vi "Test Serialize Paths.vi"(8 "error in (no error)":errorcluster) -> (0 "error out":errorcluster)   [LabVIEW 2013]
uses:
  src/Serializer/JSON Serializer/JSON Serializer.lvclass
  <vilib>/addons/_JKI Toolkits/Caraya/classes/Test/Test.lvclass
  <vilib>/addons/_JKI Toolkits/Caraya/classes/Assert/Assert.lvclass
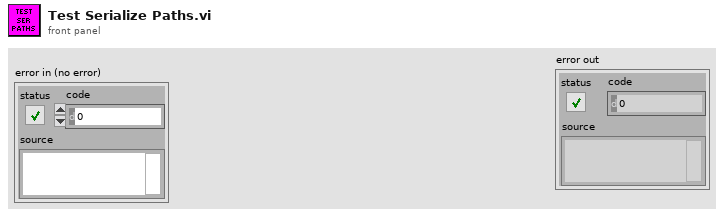
[diagram p1: front panel]
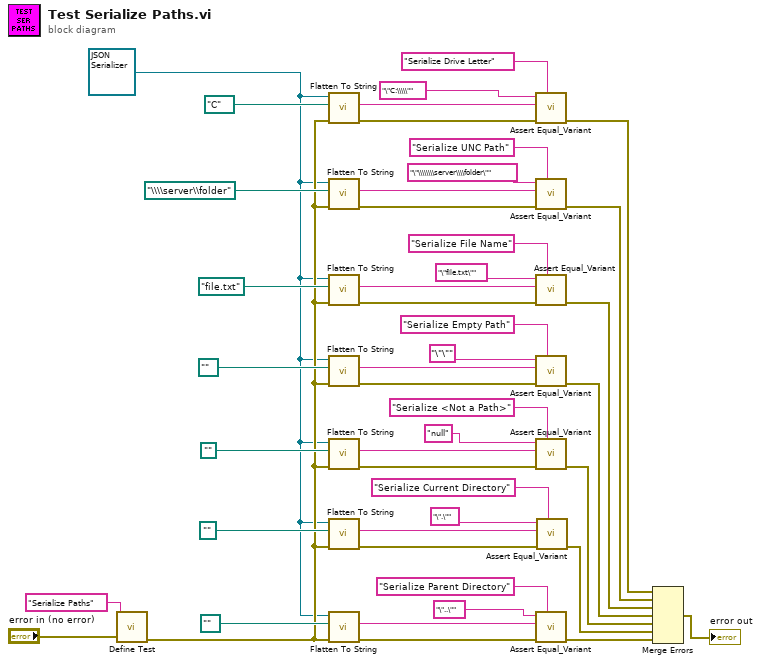
[diagram p0: block diagram]
diagram:
  w2 = refnum<class "JSON Serializer.lvclass"> refnum ("JKI JSON Serialization.lvlib:JSON Serializer.lvclass")
  n1 = call <vilib>:"Define Test.vi"("error in (no error)"="error in (no error)", "Label (VI Title)"="Serialize Paths") -> ("error out"=w3:errorcluster)  [unwired: 9 in]
  n2 = call-dynamic "Flatten To String.vi"("error in (no error)"=w3, "Variant"=path "C:/", "JSON Serializer in"=w2) -> ("error out"=w34:errorcluster, "String"=w33:string)  [unwired: 6 in, 1 out]
  n3 = call-dynamic "Flatten To String.vi"("error in (no error)"=w3, "Variant"=path "\\\\server\\folder", "JSON Serializer in"=w2) -> ("error out"=w38:errorcluster, "String"=w37:string)  [unwired: 6 in, 1 out]
  n4 = call-dynamic "Flatten To String.vi"("error in (no error)"=w3, "Variant"=path "file.txt", "JSON Serializer in"=w2) -> ("error out"=w42:errorcluster, "String"=w41:string)  [unwired: 6 in, 1 out]
  n5 = call-dynamic "Flatten To String.vi"("error in (no error)"=w3, "Variant"=path "", "JSON Serializer in"=w2) -> ("error out"=w10:errorcluster, "String"=w11:string)  [unwired: 6 in, 1 out]
  n6 = call-dynamic "Flatten To String.vi"("error in (no error)"=w3, "Variant"=path "", "JSON Serializer in"=w2) -> ("error out"=w8:errorcluster, "String"=w7:string)  [unwired: 6 in, 1 out]
  n7 = call-dynamic "Flatten To String.vi"("error in (no error)"=w3, "Variant"=path "", "JSON Serializer in"=w2) -> ("error out"=w16:errorcluster, "String"=w17:string)  [unwired: 6 in, 1 out]
  n8 = call-dynamic "Flatten To String.vi"("error in (no error)"=w3, "Variant"=path "..", "JSON Serializer in"=w2) -> ("error out"=w46:errorcluster, "String"=w45:string)  [unwired: 6 in, 1 out]
  n9 = call <vilib>:"Assert Equal_Variant.vi"("Label"="Serialize Drive Letter", "error in (no error)"=w34, "Y"=w33, "X"="\"C:\\\\\"") -> ("error out"=w26:errorcluster)  [unwired: 7 in]
  n10 = call <vilib>:"Assert Equal_Variant.vi"("Label"="Serialize UNC Path", "error in (no error)"=w38, "Y"=w37, "X"="\"\\\\\\\\server\\\\folder\"") -> ("error out"=w27:errorcluster)  [unwired: 7 in]
  n11 = call <vilib>:"Assert Equal_Variant.vi"("Label"="Serialize File Name", "error in (no error)"=w42, "Y"=w41, "X"="\"file.txt\"") -> ("error out"=w28:errorcluster)  [unwired: 7 in]
  n12 = call <vilib>:"Assert Equal_Variant.vi"("Label"="Serialize Empty Path", "error in (no error)"=w10, "Y"=w11, "X"="\"\"") -> ("error out"=w9:errorcluster)  [unwired: 7 in]
  n13 = call <vilib>:"Assert Equal_Variant.vi"("Label"="Serialize <Not a Path>", "error in (no error)"=w8, "Y"=w7, "X"="null") -> ("error out"=w1:errorcluster)  [unwired: 7 in]
  n14 = call <vilib>:"Assert Equal_Variant.vi"("Label"="Serialize Parent Directory", "error in (no error)"=w46, "Y"=w45, "X"="\"..\"") -> ("error out"=w29:errorcluster)  [unwired: 7 in]
  n15 = call <vilib>:"Assert Equal_Variant.vi"("Label"="Serialize Current Directory", "error in (no error)"=w16, "Y"=w17, "X"="\".\"") -> ("error out"=w15:errorcluster)  [unwired: 7 in]
  n16 = Merge Errors(w26, w27, w28, w9, w1, w15, w29) -> (→"error out":errorcluster)
